vi "sv_Initialize Swept Measurements Array.vi"(4 "harmonic mapping":u32[](array[numeric]), 6 "maximum THD harmonic":u32, 8 "AI freq index":i32, 9 "RMS level":bool, 10 "# of points":i32, 11 "measurements in":T1 {"scaled response magnitude" format="%.3f"; "Harm[]" format="%.2f"; "THD" format="%.2f"; "Im [response]" format="%.2f"; "Re [response]" format="%.2f"; "Im [stimulus]" format="%.2f"; "Re [stimulus]" format="%.2f"; "RMS response" format="%.2f"; "RMS stimulus" format="%.2f"}) -> (1 "dup RMS level":bool, 3 "measurements out":T1 {"scaled response magnitude" format="%.3f"; "Harm[]" format="%.2f"; "THD" format="%.2f"; "Im [response]" format="%.2f"; "Re [response]" format="%.2f"; "Im [stimulus]" format="%.2f"; "Re [stimulus]" format="%.2f"; "RMS response" format="%.2f"; "RMS stimulus" format="%.2f"})   [LabVIEW 2017, in "SoundVib_SweptSine.lvlib"]
uses:
  <vilib>/addons/Sound and Vibration/svt_Swept Sine/SoundVib_SweptSine.lvlib
  <vilib>/addons/Sound and Vibration/svt_Swept Sine/subVIs/sv_Swept Sine Measurements.ctl
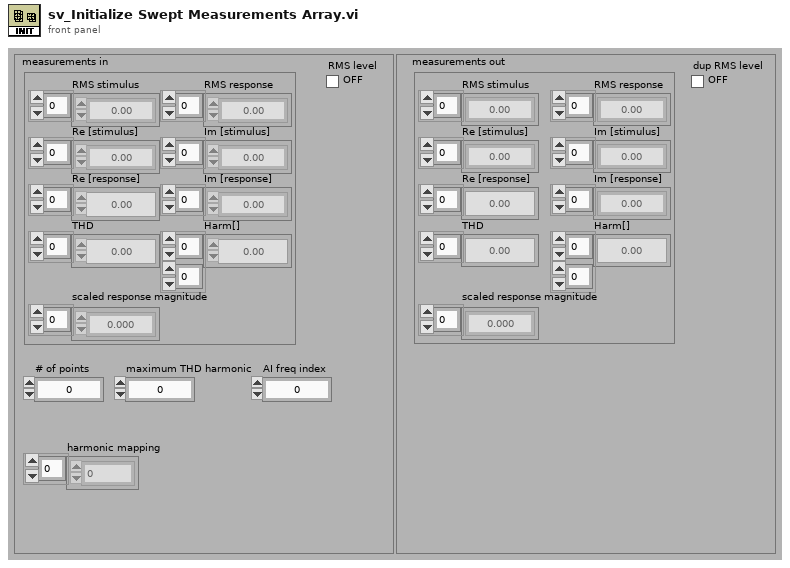
[diagram p1: front panel]
types:
  T1 = typedef "SoundVib_SweptSine.lvlib/sv_Swept Sine Measurements.ctl" = cluster{"RMS stimulus":dbl[], "RMS response":dbl[], "Re [stimulus]":dbl[], "Im [stimulus]":dbl[], "Re [response]":dbl[], "Im [response]":dbl[], "THD":dbl[], "Harm[]":dbl[][], "scaled response magnitude":dbl[]}
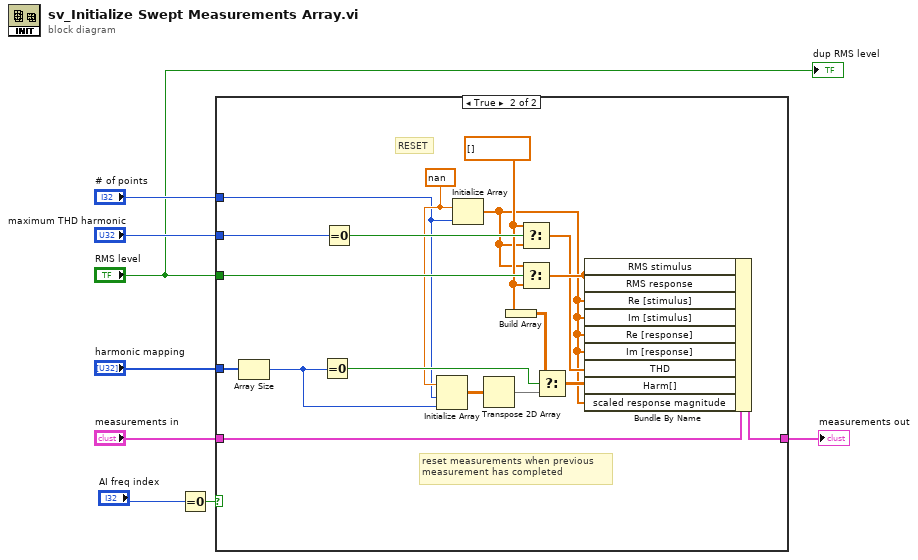
[diagram p0: block diagram]
diagram:
  n1 = Equal To 0?(x="AI freq index") -> (x = 0?=w2:bool)
  n2 = case shown="True" w2 {
    tunnel: "RMS level" -> [_ w27]
    tunnel: "measurements in" -> [w9 w26]
    tunnel: [w9 w25] -> w7
    tunnel: "# of points" -> [_ w13]
    tunnel: "maximum THD harmonic" -> [_ w12]
    tunnel: "harmonic mapping" -> [_ w11]
    frame False {
    }
    frame True {
      w16 = dbl[] [] ("RMS stimulus")
      w15 = nan ("element")
      # "reset measurements when previous \nmeasurement has completed"
      # "RESET"
      n3 = Array Size(array=w11) -> (size(s)=w10:i32)
      n4 = Equal To 0?(x=w10) -> (x = 0?=w23:bool)
      n5 = Equal To 0?(x=w12) -> (x = 0?=w24:bool)
      n6 = Initialize Array(w15, w13, w10) -> (w20:dbl[][])
      n7 = Initialize Array(w15, w13) -> (w14:dbl[])
      n8 = Transpose 2D Array(2D array=w20) -> (transposed array=w19:dbl[][])
      n9 = Build Array(w16) -> (w21:dbl[][])
      n10 = Select(t=w16, s=w24, f=w14) -> (s? t:f=w17:dbl[])
      n11 = Select(t=w14, s=w27, f=w16) -> (s? t:f=w18:dbl[])
      n12 = Select(t=w21, s=w23, f=w19) -> (s? t:f=w22:dbl[][])
      n13 = Bundle By Name(cluster=w26, "RMS stimulus"=w18, "RMS response"=w18, "Re [stimulus]"=w14, "Im [stimulus]"=w14, "Re [response]"=w14, "Im [response]"=w14, "THD"=w17, "Harm[]"=w22, "scaled response magnitude"=w14) -> (w25:T1)
    }
  }
  "measurements out" <- w7
  "dup RMS level" <- "RMS level"
